vi "TEMTE.vi"(0 "Type and run direction":T2=enum."ASCII", 2 "LS Multiplier":dbl=1.1, 5 "Font refnum":refnum<k24>, 7 "Alignment":T1, 9 "Text":string, 11 "error in (no error)":errorcluster) -> (4 "Paragraph":refnum<k24>, 15 "error out":errorcluster)   [LabVIEW 2019]
doc: "Developed by Jean-Marc Simard\nCopyright © 2012, Exaprom Inc.\nAll rights reserved.\nLicense: BSD\n\nWith iTextSharp 4.1.6 (http://itextsharp.sourceforge.net)\nunder Mozilla Public License Version 1.1\n(http://www.mozilla.org/MPL/MPL-1.1.html)"
uses:
  <userlib>/Exaprom PDF/Controls/Text Controls/Unicode/Type and run direction.ctl
  C:/Program Files/National Instruments/LabVIEW 2019/user.lib/Exaprom PDF/DLL/itextsharp.dll
  DLL/itextsharp.dll
  <userlib>/Exaprom PDF/Controls/Header, Footer and Watermark Controls/Header footer horiz alignment.ctl
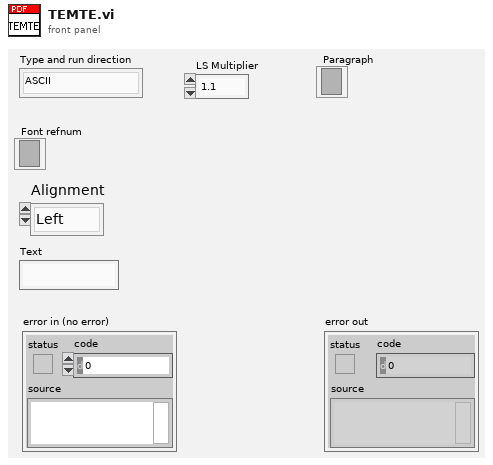
[diagram p1: front panel]
types:
  T1 = typedef "Header footer horiz alignment.ctl" = enum16{"Left", "Center", "Right"}
  T2 = typedef "Type and run direction.ctl" = enum16{"Select", "ASCII", "UTF-16", "UTF-16 (default)", "UTF-16 (LTR)", "UTF-16 (RTL)"}
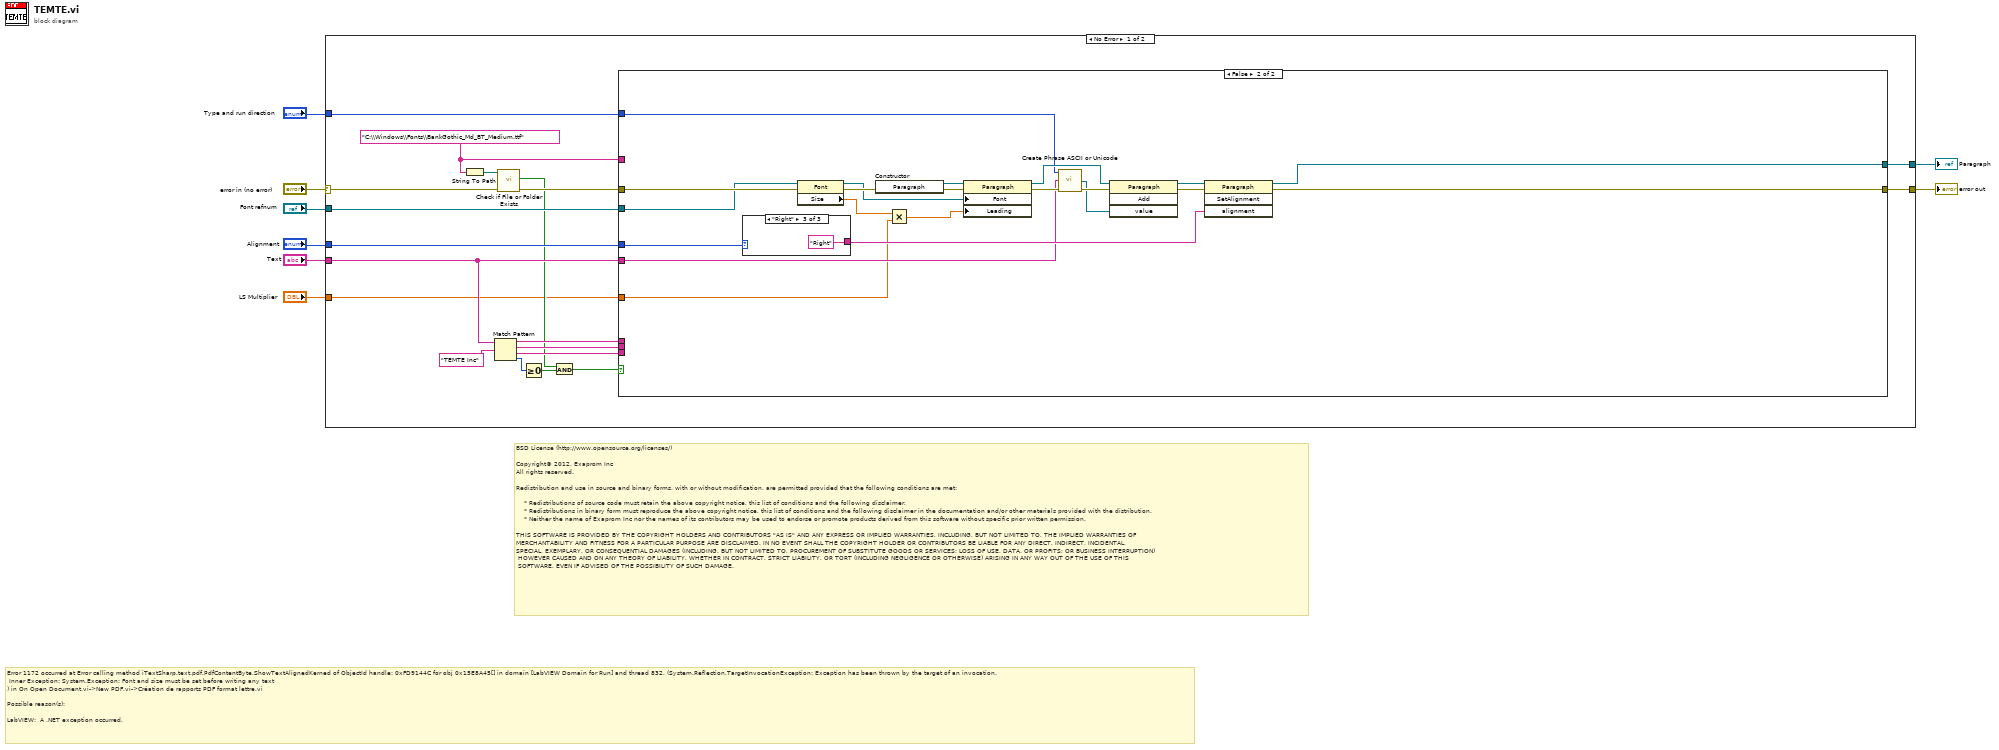
[diagram p0: block diagram]
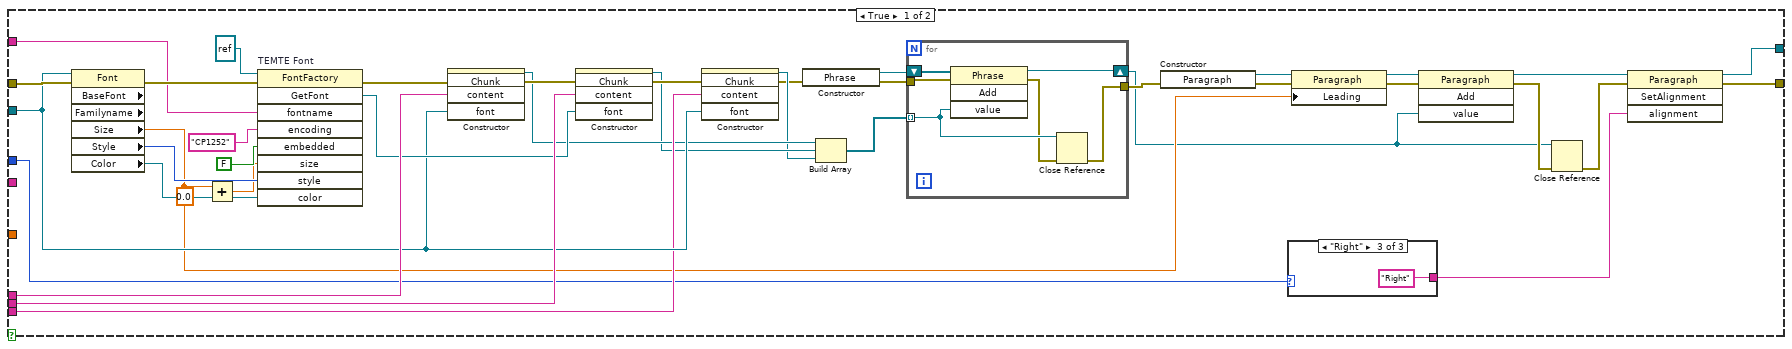
[diagram p2: hidden frame]
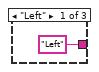
[diagram p3: hidden frame]
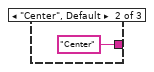
[diagram p4: hidden frame]
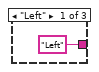
[diagram p5: hidden frame]
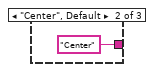
[diagram p6: hidden frame]
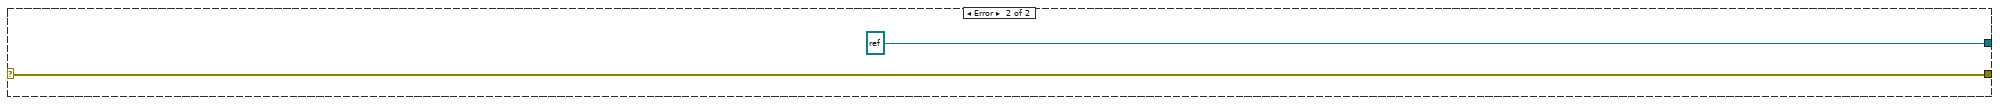
[diagram p7: hidden frame]
diagram:
  # "Error 1172 occurred at Error calling method iTextSharp.text.pdf.PdfContentByte.ShowTextAlignedKerned of ObjectId handle: 0xFD9144C for obj 0x15E8A45[] in domain [LabVIEW Domain for Run] and thread 832, (System.Reflection.TargetInvocationException: Exception has been thrown by the target of an invocation.\n\tInner Exception: System.Exception: Font and size must be set before writing any text\n) in On Open Document.vi->New PDF.vi->Création de rapports PDF format lettre.vi\n\nPossible reason(s):\n\nLabVIEW:  A .NET exception occurred."
  # "BSD License (http://www.opensource.org/licenses/)\n\nCopyright© 2012, Exaprom Inc\nAll rights reserved.\n\nRedistribution and use in source and binary forms, with or without modification, are permitted provided that the following conditions are met:\n\n    * Redistributions of source code must retain the above copyright notice, this list of conditions and the following disclaimer.\n    * Redistributions in binary form must reproduce the above copyright notice, this list of conditions and the following disclaimer in the documentation and/or other materials provided with the distribution.\n    * Neither the name of Exaprom Inc nor the names of its contributors may be used to endorse or promote products derived from this software without specific prior written permission.\n\nTHIS SOFTWARE IS PROVIDED BY THE COPYRIGHT HOLDERS AND CONTRIBUTORS \"AS IS\" AND ANY EXPRESS OR IMPLIED WARRANTIES, INCLUDING, BUT NOT LIMITED TO, THE IMPLIED WARRANTIES OF \nMERCHANTABILITY AND FITNESS FOR A PARTICULAR PURPOSE ARE DISCLAIMED. IN NO EVENT SHALL THE COPYRIGHT HOLDER OR CONTRIBUTORS BE LIABLE FOR ANY DIRECT, INDIRECT, INCIDENTAL,\nSPECIAL, EXEMPLARY, OR CONSEQUENTIAL DAMAGES (INCLUDING, BUT NOT LIMITED TO, PROCUREMENT OF SUBSTITUTE GOODS OR SERVICES; LOSS OF USE, DATA, OR PROFITS; OR BUSINESS INTERRUPTION)\n HOWEVER CAUSED AND ON ANY THEORY OF LIABILITY, WHETHER IN CONTRACT, STRICT LIABILITY, OR TORT (INCLUDING NEGLIGENCE OR OTHERWISE) ARISING IN ANY WAY OUT OF THE USE OF THIS\n SOFTWARE, EVEN IF ADVISED OF THE POSSIBILITY OF SUCH DAMAGE."
  n1 = case shown="No Error" "error in (no error)" {
    selector: "error in (no error)" -> [w16 w101]
    tunnel: [w27 w101] -> w8
    tunnel: [w26 refnum<k24> refnum ("new reference")] -> w6
    tunnel: "Type and run direction" -> [w25 _]
    tunnel: "Font refnum" -> [w24 _]
    tunnel: "Alignment" -> [w23 _]
    tunnel: "Text" -> [w22 _]
    tunnel: "LS Multiplier" -> [w9 _]
    frame No Error {
      w10 = "C:\\Windows\\Fonts\\BankGothic_Md_BT_Medium.ttf"
      n2 = String To Path(string=w10) -> (path=w14:path)
      n3 = Match Pattern(string=w22, regular expression="TEMTE Inc") -> (before substring=w19:string, match substring=w20:string, after substring=w18:string, offset past match=w17:i32)  [unwired: 1 in]
      n4 = call <vilib>:"Check if File or Folder Exists.vi"("error in (no error)"=w16, "path"=w14) -> ("error out"=w15:errorcluster, "file or folder exists?"=w12:bool)  [unwired: 7 in, 1 out]
      n5 = Greater Or Equal To 0?(x=w17) -> (x >= 0?=w13:bool)
      n6 = And(x=w12, y=w13) -> (x .and. y?=w11:bool)
      n7 = case shown="False" w11 {
        tunnel: [w35 w85] -> w27
        tunnel: [w31 w84] -> w26
        tunnel: w15 -> [w65 w83]
        tunnel: w25 -> [_ w82]
        tunnel: w24 -> [w52 w81]
        tunnel: w23 -> [w30 w80]
        tunnel: w22 -> [_ w79]
        tunnel: w20 -> [w55 _]
        tunnel: w19 -> [w57 _]
        tunnel: w18 -> [w51 _]
        tunnel: w10 -> [w63 _]
        tunnel: w9 -> [_ w78]
        frame True {
          n8 = property class="Font" props=["BaseFont", "Familyname", "Size", "Style", "Color"](reference=w52, error in=w65) -> (error out=w64:errorcluster, "Size"=w40:sgl, "Style"=w62:i32, "Color"=w61:refnum<k24>)  [unwired: 3 out]
          n9 = Add(x=w40, y=sgl 0.0) -> (x+y=w29:sgl)
          n10 = invoke on="TEMTE Font" class="FontFactory" method="GetFont"(reference=refnum<k24> refnum, error in=w64, "fontname"=w63, "encoding"="CP1252", "embedded"=FALSE, "size"=w29, "style"=w62, "color"=w61) -> (error out=w58:errorcluster, "GetFont"=w54:refnum<k24>)  [unwired: 1 in, 7 out]
          n11 = constructor class="Chunk"(error in=w58, "content"=w57, "font"=w52) -> (reference out=w50:refnum<k24>, error out=w56:errorcluster)  [unwired: 2 in, 3 out]
          n12 = constructor class="Chunk"(error in=w56, "content"=w55, "font"=w54) -> (reference out=w49:refnum<k24>, error out=w53:errorcluster)  [unwired: 2 in, 3 out]
          n13 = constructor class="Chunk"(error in=w53, "content"=w51, "font"=w52) -> (reference out=w48:refnum<k24>, error out=w47:errorcluster)  [unwired: 2 in, 3 out]
          n14 = constructor class="Phrase"(error in=w47) -> (reference out=w45:refnum<k24>, error out=w46:errorcluster)  [unwired: 2 in, 1 out]
          n15 = Build Array(w50, w49, w48) -> (w44:refnum<k24>[])
          n16 = for {
            shift-right: [w74] -> w38
            shift-left: w45 -> [w75]
            tunnel: w46 -> [w71]
            tunnel: w44 -> [w73] mode=indexing
            tunnel: [w70] -> w41
            n17 = invoke class="Phrase" method="Add"(reference=w75, error in=w71, "value"=w73) -> (reference out=w74:refnum<k24>, error out=w72:errorcluster)  [unwired: 1 in, 2 out]
            n18 = Close Reference(reference=w73, error in (no error)=w72) -> (error out=w70:errorcluster)
          }
          n19 = constructor class="Paragraph"(error in=w41) -> (reference out=w42:refnum<k24>, error out=w43:errorcluster)  [unwired: 2 in, 1 out]
          n20 = case shown="\"Right\"" w30 {
            tunnel: ["Left" "Center" "Right"] -> w32
            frame "Left" {
            }
            frame "Center", Default {
            }
            frame "Right" {
            }
          }
          n21 = property class="Paragraph"(reference=w42, error in=w43, "Leading"=w40) -> (reference out=w36:refnum<k24>, error out=w37:errorcluster)
          n22 = invoke class="Paragraph" method="Add"(reference=w36, error in=w37, "value"=w38) -> (reference out=w33:refnum<k24>, error out=w39:errorcluster)  [unwired: 1 in, 2 out]
          n23 = Close Reference(reference=w38, error in (no error)=w39) -> (error out=w34:errorcluster)
          n24 = invoke class="Paragraph" method="SetAlignment"(reference=w33, error in=w34, "alignment"=w32) -> (reference out=w31:refnum<k24>, error out=w35:errorcluster)  [unwired: 1 in, 2 out]
        }
        frame False {
          n25 = case shown="\"Right\"" w80 {
            tunnel: ["Left" "Center" "Right"] -> w96
            frame "Left" {
            }
            frame "Center", Default {
            }
            frame "Right" {
            }
          }
          n26 = property class="Font"(reference=w81, error in=w83) -> (reference out=w92:refnum<k24>, error out=w95:errorcluster, "Size"=w77:sgl)
          n27 = constructor class="Paragraph"(error in=w95) -> (reference out=w93:refnum<k24>, error out=w94:errorcluster)  [unwired: 2 in, 1 out]
          n28 = Multiply(x=w77, y=w78) -> (x*y=w76:dbl)
          n29 = property class="Paragraph"(reference=w93, error in=w94, "Font"=w92, "Leading"=w76) -> (reference out=w89:refnum<k24>, error out=w88:errorcluster)
          n30 = call <userlib>:"Create Phrase ASCII or Unicode.vi"("Character type"=w82, "Text"=w79, "error in (no error)"=w88) -> ("Phrase refnum"=w86:refnum<k24>, "error out"=w87:errorcluster)  [unwired: 10 in, 1 out]
          n31 = invoke class="Paragraph" method="Add"(reference=w89, error in=w87, "value"=w86) -> (reference out=w91:refnum<k24>, error out=w90:errorcluster)  [unwired: 1 in, 2 out]
          n32 = invoke class="Paragraph" method="SetAlignment"(reference=w91, error in=w90, "alignment"=w96) -> (reference out=w84:refnum<k24>, error out=w85:errorcluster)  [unwired: 1 in, 2 out]
        }
      }
    }
    frame Error {
    }
  }
  "error out" <- w8
  "Paragraph" <- w6
